vi "Command Toggle Intake Rotation.vi"(2 "Robot System Functions In":T1, 3 "Startup":bool, 4 "String Parameter":string, 5 "Cmd Parameter 3":dbl, 6 "Cmd Parameter 2":dbl, 7 "Cmd Parameter 1":dbl) -> (0 "Robot System Functions Out":T1, 1 "Completed":bool)   [LabVIEW 2016]
uses:
  Subsystems/All Robot Commands.ctl
  Subsystems/Drive and Climb SS/Drive + Climb Commands 2017.ctl
  Subsystems/Gear Delivery SS/Gear Delivery Commands.ctl
  Subsystems/Conveyor and Shooter SS/Conveyor and Shooter Commands.ctl
  Subsystems/Ball Intake SS/Ball Intake Commands.ctl
  Command Execution State.ctl
panel:
  # "Sample robot\ncontrol output.\nReplace with \nactual teleop \ncontrol signal \nstructure."
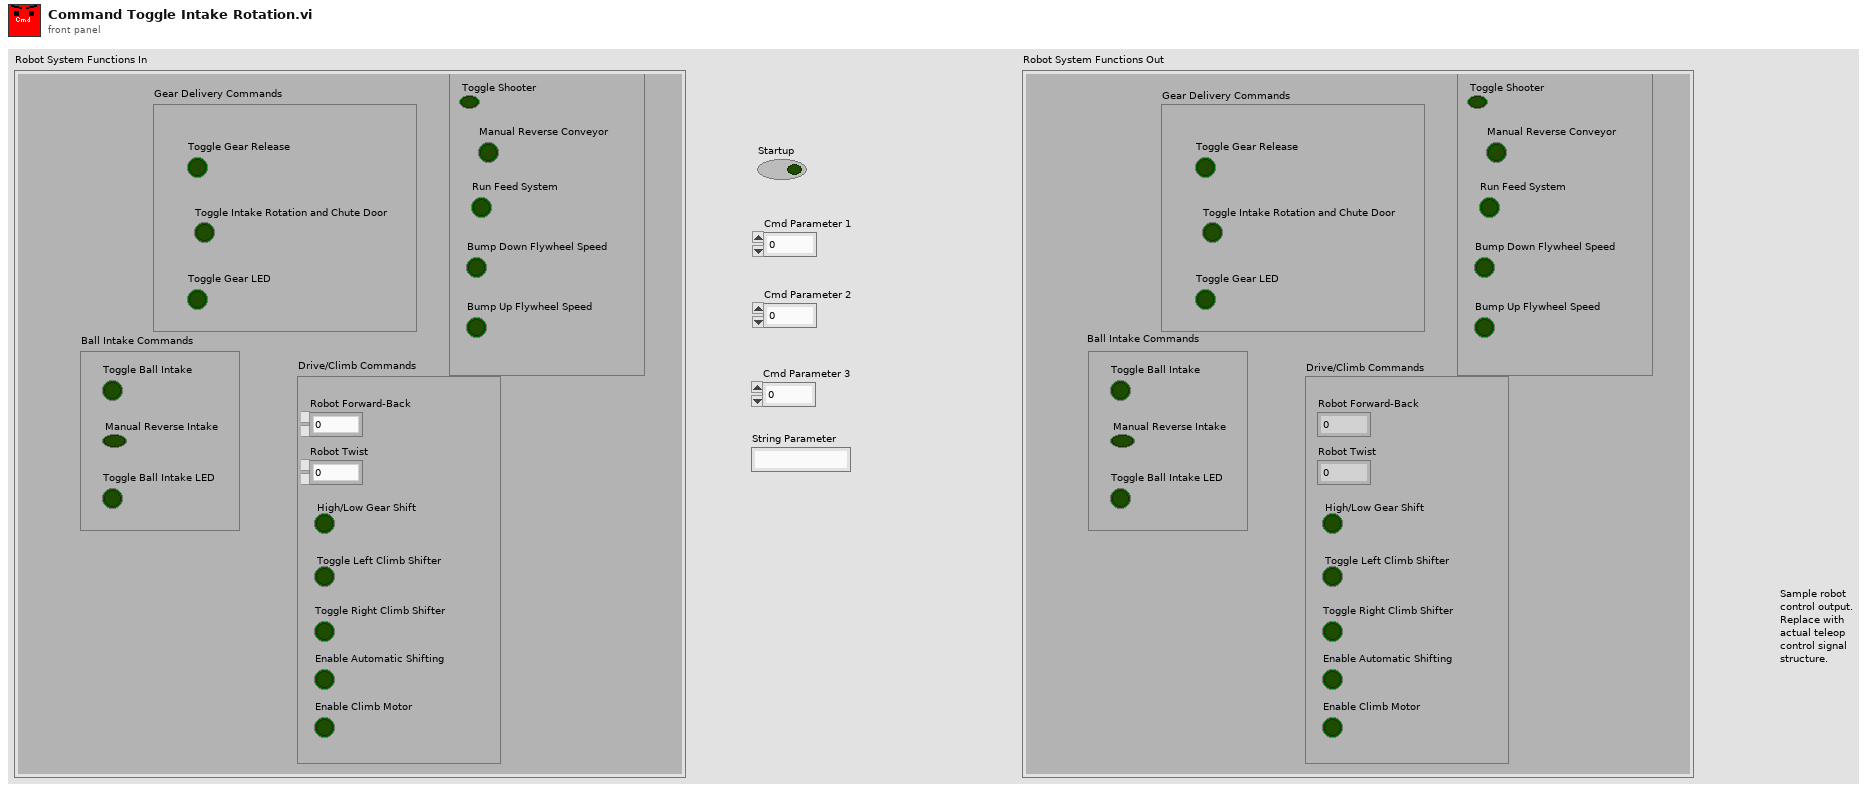
[diagram p1: front panel]
types:
  T1 = typedef "All Robot Commands.ctl" = cluster{"Drive/Climb Commands":T2, "Gear Delivery Commands":T3, "Shooter and Conveyor Commands":T4, "Ball Intake Commands":T5}
  T2 = typedef "Drive + Climb Commands 2017.ctl" = cluster{"Robot Forward-Back":dbl, "Robot Twist":dbl, "High/Low Gear Shift":bool, "Toggle Left Climb Shifter":bool, "Toggle Right Climb Shifter":bool, "Enable Automatic Shifting":bool, "Enable Climb Motor ":bool}
  T3 = typedef "Gear Delivery Commands.ctl" = cluster{"Toggle Gear Release":bool, "Toggle Intake Rotation and Chute Door":bool, "Toggle Gear LED":bool}
  T4 = typedef "Conveyor and Shooter Commands.ctl" = cluster{"Toggle Shooter":bool, "Manual Reverse Conveyor":bool, "Run Feed System":bool, "Bump Down Flywheel Speed":bool, "Bump Up Flywheel Speed":bool}
  T5 = typedef "Ball Intake Commands.ctl" = cluster{"Toggle Ball Intake":bool, "Manual Reverse Intake":bool, "Toggle Ball Intake LED":bool}
  T6 = typedef "Command Execution State.ctl" = enum16{"Initialize", "Execute", "Finish"}
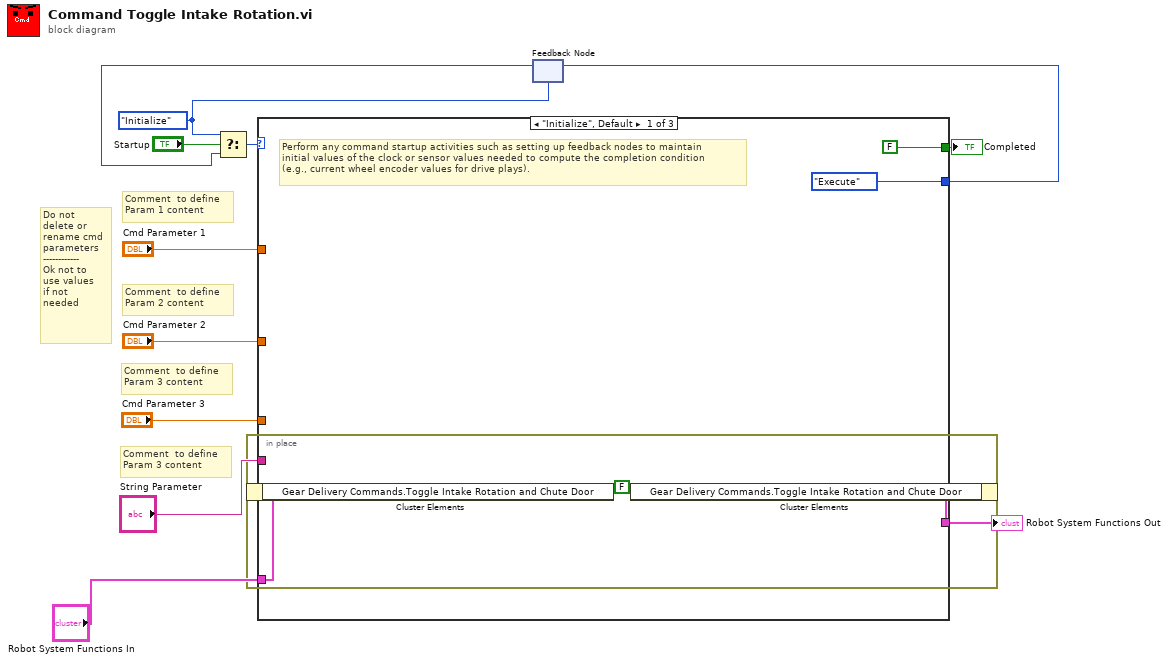
[diagram p0: block diagram]
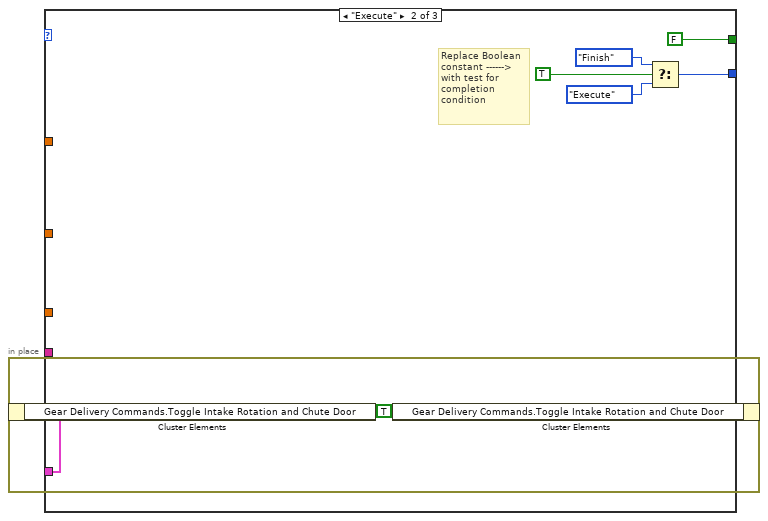
[diagram p2: hidden frame]
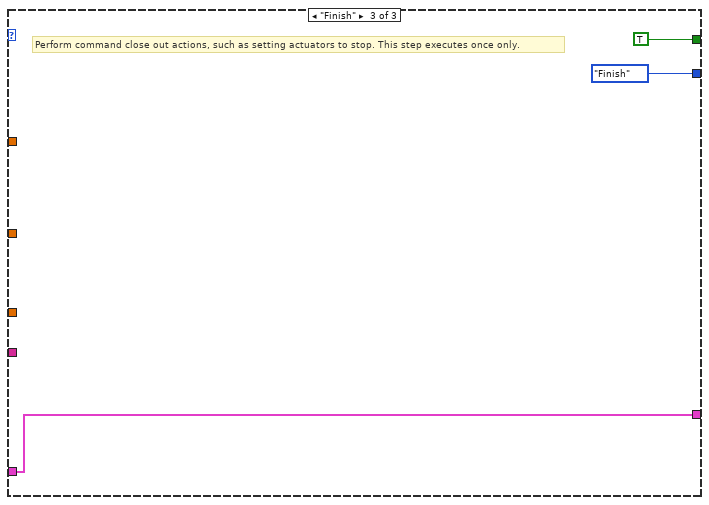
[diagram p3: hidden frame]
diagram:
  w7 = Command_Execution_State."Initialize" ("Play State")
  # "Comment  to define\nParam 3 content"
  # "Comment  to define\nParam 3 content"
  # "Do not \ndelete or\nrename cmd\nparameters\n------------\nOk not to \nuse values\nif not \nneeded"
  # "Comment  to define\nParam 2 content"
  # "Comment  to define\nParam 1 content"
  n1 = feedback #1(w7) -> (w8:T6)
  n2 = Select(t=w7, s="Startup", f=w8) -> (s? t:f=w12:T6)
  n3 = case shown="\"Initialize\", Default" w12 {
    tunnel: [FALSE FALSE TRUE] -> w10
    tunnel: [Command_Execution_State."Execute" ("Play State") w22 Command_Execution_State."Finish" ("f")] -> w9
    tunnel: "Cmd Parameter 1" -> [_ _ _]
    tunnel: "Cmd Parameter 2" -> [_ _ _]
    tunnel: [w13 w18 w26] -> w4
    tunnel: "Robot System Functions In" -> [w14 w19 w26]
    tunnel: "Cmd Parameter 3" -> [_ _ _]
    tunnel: "String Parameter" -> [_ _ _]
    frame "Initialize", Default {
      # "Perform any command startup activities such as setting up feedback nodes to maintain \ninitial values of the clock or sensor values needed to compute the completion condition\n(e.g., current wheel encoder values for drive plays)."
      n4 = in-place {
        n5 = in-place-cluster #2(w14) -> ()  [unwired: 1 out]
        n6 = in-place-cluster #2("Gear Delivery Commands.Toggle Intake Rotation and Chute Door"=FALSE) -> (w13:T1)
      }
    }
    frame "Execute" {
      # "Replace Boolean\nconstant ------>\nwith test for \ncompletion \ncondition"
      n7 = in-place {
        n8 = in-place-cluster #3(w19) -> ()  [unwired: 1 out]
        n9 = in-place-cluster #3("Gear Delivery Commands.Toggle Intake Rotation and Chute Door"=TRUE ("Gear Delivery Commands.Toggle Intake Rotation")) -> (w18:T1)
      }
      n10 = Select(t=Command_Execution_State."Finish" ("Play State"), s=TRUE, f=Command_Execution_State."Execute") -> (s? t:f=w22:T6)
    }
    frame "Finish" {
      # "Perform command close out actions, such as setting actuators to stop. This step executes once only."
    }
  }
  "Completed" <- w10
  "Robot System Functions Out" <- w4
  n11 = feedback-in #1(w9) -> ()
